vi "Add Alias Folder.vi"(7 "Overwrite Existing?":bool=TRUE, 8 "error in (no error)":errorcluster, 9 "Alias Folder Settings":T1, 10 "Base Node Path":string, 11 "SysDef Ref":T2) -> (0 "error out":errorcluster, 2 "New Node Path":string, 3 "SysDef Ref Out":T2)   [LabVIEW 2019, in "Simple SysDef API.lvlib"]
uses:
  <userlib>/SimpleSysDef/Simple SysDef API.lvlib
  <userlib>/SimpleSysDef/_SubVIs/System Definition Reference.ctl
  NationalInstruments.VeriStand.SystemDefinitionAPI
  <userlib>/SimpleSysDef/_SubVIs/Add Folder_Settings.ctl
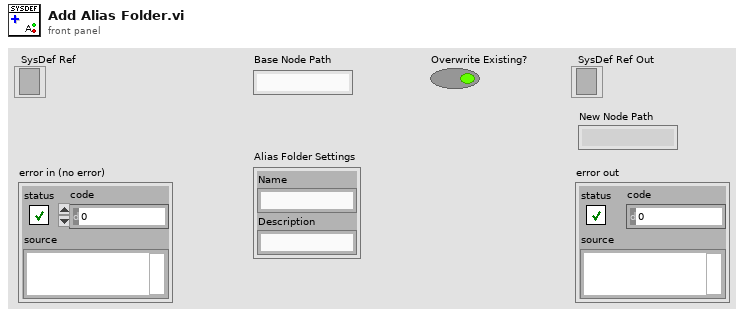
[diagram p1: front panel]
types:
  T1 = typedef "Simple SysDef API.lvlib/Add Folder_Settings.ctl" = cluster{"Name":string, "Description":string}
  T2 = typedef "Simple SysDef API.lvlib/System Definition Reference.ctl" = refnum<k24>
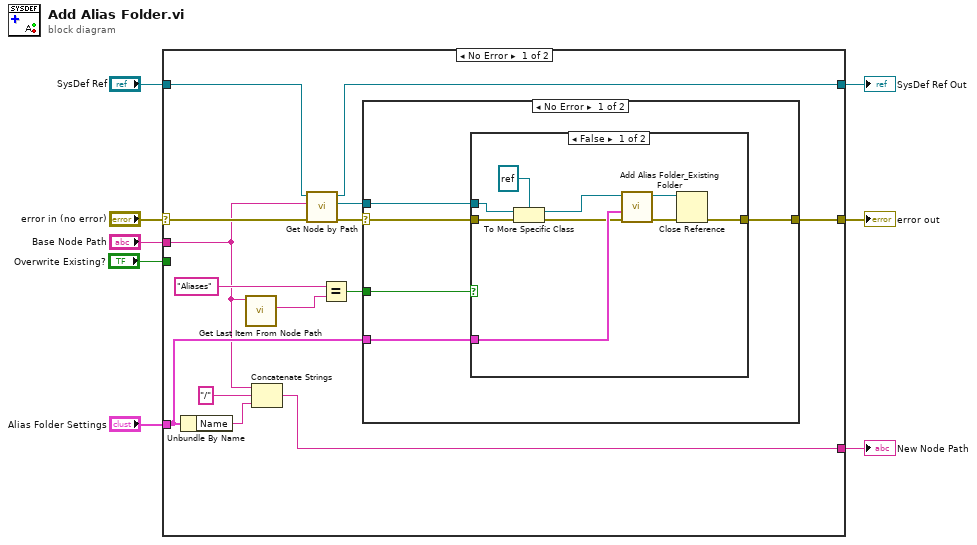
[diagram p0: block diagram]
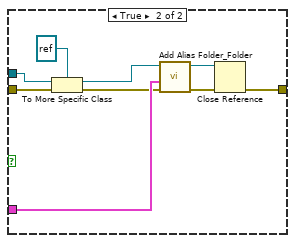
[diagram p2: hidden frame]
diagram:
  n1 = case shown="No Error" "error in (no error)" {
    selector: "error in (no error)" -> [w12 w48]
    tunnel: [w20 w48] -> w7
    tunnel: "SysDef Ref" -> [w14 w47]
    tunnel: [w13 w47] -> w5
    tunnel: "Base Node Path" -> [w10 _]
    tunnel: "Overwrite Existing?" -> [_ _]
    tunnel: "Alias Folder Settings" -> [w18 _]
    tunnel: [w19 _] -> w1
    frame No Error {
      n2 = Unbundle By Name(w18) -> ("Name"=w21:string)
      n3 = call <userlib>:"Get Last Item From Node Path.vi"("Name"=w10) -> ("Last Item"=w15:string)  [unwired: 9 in, 1 out]
      n4 = Concatenate Strings(w10, "/" ("string"), w21) -> (w19:string)
      n5 = call <userlib>:"Get Node by Path.vi"("error in (no error)"=w12, "System Definition Node Path"=w10, "SysDef Ref"=w14) -> ("error out"=w11:errorcluster, "Node Ref"=w9:refnum<k24>, "SysDef Ref Out"=w13:T2)  [unwired: 6 in]
      n6 = Equal?(x="Aliases", y=w15) -> (x = y?=w16:bool)
      n7 = case shown="No Error" w11 {
        selector: w11 -> [w26 w46]
        tunnel: [w25 w46] -> w20
        tunnel: w9 -> [w27 _]
        tunnel: w18 -> [w24 _]
        tunnel: w16 -> [w23 _]
        frame No Error {
          n8 = case shown="False" w23 {
            tunnel: w27 -> [w36 w45]
            tunnel: w26 -> [w35 w44]
            tunnel: [w34 w43] -> w25
            tunnel: w24 -> [w31 w40]
            frame False {
              n9 = To More Specific Class(target class=refnum<k24> refnum ("Node Ref"), reference=w36, error in=w35) -> (specific class reference=w32:refnum<k24>, error out=w30:errorcluster)
              n10 = call <userlib>:"Add Alias Folder_Existing Folder.vi"("error in (no error)"=w30, "Alias Folder Settings"=w31, "Alias Folder Ref"=w32) -> ("error out"=w28:errorcluster, "Alias Folder Ref out"=w29:refnum<k24>)  [unwired: 7 in]
              n11 = Close Reference(reference=w29, error in (no error)=w28) -> (error out=w34:errorcluster)
            }
            frame True {
              n12 = To More Specific Class(target class=refnum<k24> refnum ("Node Ref"), reference=w45, error in=w44) -> (specific class reference=w41:refnum<k24>, error out=w39:errorcluster)
              n13 = call <userlib>:"Add Alias Folder_Folder.vi"("error in (no error)"=w39, "Alias Folder Settings"=w40, "Alias Folder Ref"=w41) -> ("error out"=w38:errorcluster, "Alias Folder Ref out"=w37:refnum<k24>)  [unwired: 7 in]
              n14 = Close Reference(reference=w37, error in (no error)=w38) -> (error out=w43:errorcluster)
            }
          }
        }
        frame Error {
        }
      }
    }
    frame Error {
    }
  }
  "SysDef Ref Out" <- w5
  "error out" <- w7
  "New Node Path" <- w1
